vi "transform.vi"(9 "Demodulated signals":waveform(sgl)[][](array[waveform]), 11 "Configuration":T2) -> (0 "Sum amplitudes":sgl[][](array[numeric]), 1 "Match error":waveform(sgl)[](array[waveform]), 3 "XYZ out":T1(array[cluster]), 4 "Axis positions":sgl[][](array[numeric]))   [LabVIEW 2012]
uses:
  initialization/configuration.ctl
  initialization/asap_calibration.ctl
  <vilib>/Analysis/Matrix/Datatypes/RealMatrix.ctl
  <vilib>/Analysis/Matrix/NI_Matrix.lvlib
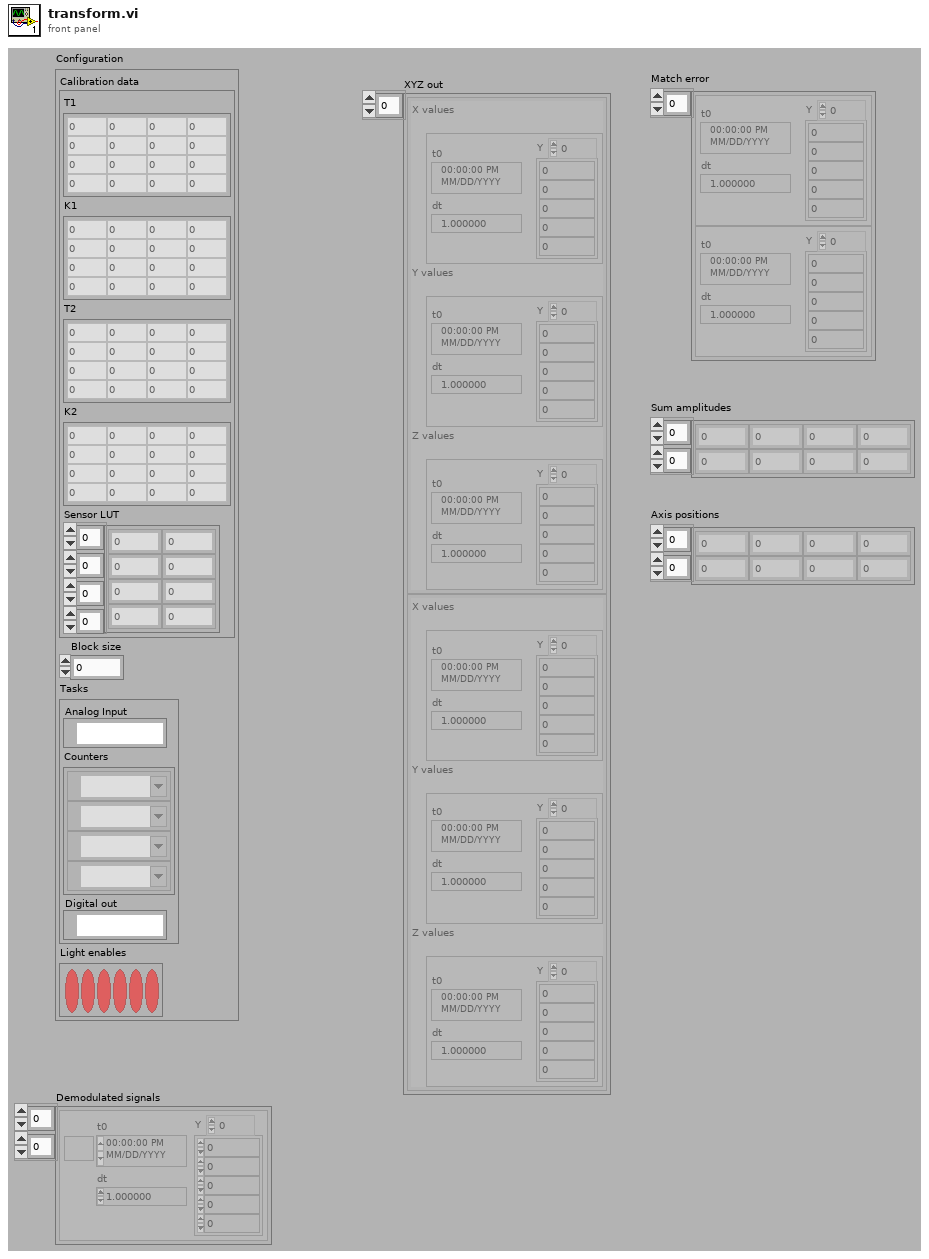
[diagram p1: front panel]
types:
  T1 = cluster{"X values":waveform(sgl), "Y values":waveform(sgl), "Z values":waveform(sgl)}[]
  T2 = typedef "configuration.ctl" = cluster{"Calibration data":T3, "Block size":i32, "Tasks":cluster{"Analog Input":refnum<k21>, "Counters":refnum<k21>[], "Digital out":refnum<k21>}, "Light enables":bool[]}
  T3 = typedef "asap_calibration.ctl" = cluster{"T1":T4, "K1":T4, "T2":T4, "K2":T4, "Sensor LUT":sgl[][][][]}
  T4 = typedef "NI_Matrix.lvlib/RealMatrix.ctl" = dbl[][]
  T5 = cluster{"X values":waveform(dbl), "Y values":waveform(dbl), "Z values":waveform(dbl)}
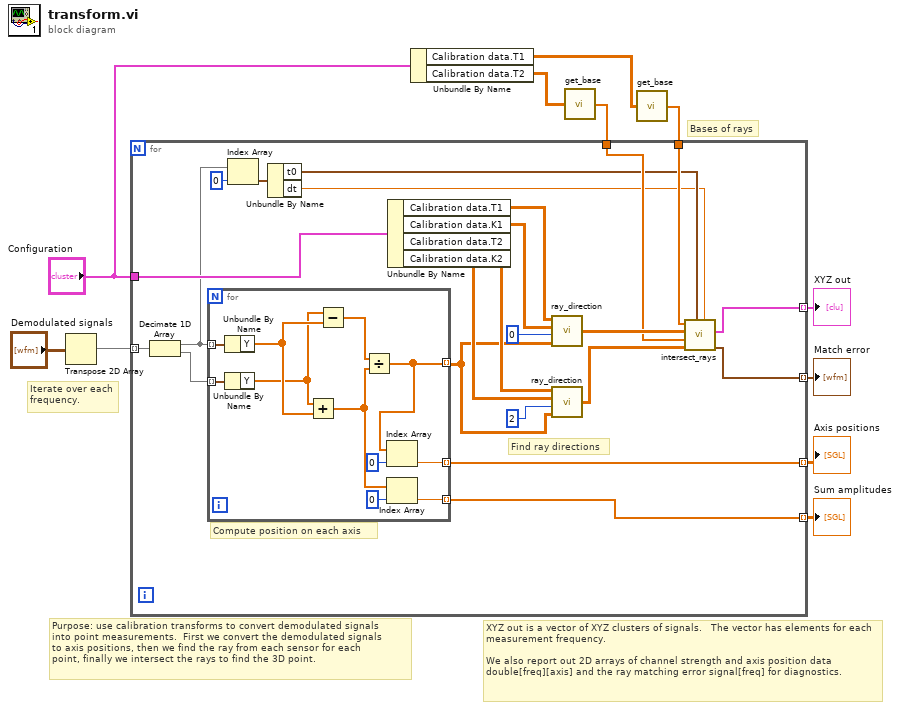
[diagram p0: block diagram]
diagram:
  # "Bases of rays"
  # "Purpose: use calibration transforms to convert demodulated signals\ninto point measurements.  First we convert the demodulated signals\nto axis positions, then we find the ray from each sensor for each\npoint, finally we intersect the rays to find the 3D point."
  # "XYZ out is a vector of XYZ clusters of signals.   The vector has elements for each\nmeasurement frequency. \n\nWe also report out 2D arrays of channel strength and axis position data double[freq][axis] and the ray matching error signal[freq] for diagnostics."
  # "Iterate over each\nfrequency."
  n1 = Transpose 2D Array(2D array="Demodulated signals") -> (transposed array=w10:waveform(sgl)[][])
  n2 = Unbundle By Name("Configuration") -> ("Calibration data.T1"=w5:T4, "Calibration data.T2"=w3:T4)
  n3 = call "get_base.vi"("T"=w3) -> ("Array"=w2:dbl[])
  n4 = call "get_base.vi"("T"=w5) -> ("Array"=w4:dbl[])
  n5 = for {
    tunnel: w10 -> [w34] mode=indexing
    tunnel: "Configuration" -> [w31]
    tunnel: [w32] -> w9 mode=indexing
    tunnel: w4 -> [w20]
    tunnel: w2 -> [w18]
    tunnel: [w14] -> w7 mode=indexing
    tunnel: [w13] -> w6 mode=indexing
    tunnel: [w12] -> w1 mode=indexing
    # "Find ray directions"
    # "Compute position on each axis"
    n6 = Decimate 1D Array(w34) -> (w30:waveform(sgl)[], w33:waveform(sgl)[])
    n7 = for {
      tunnel: [w36] -> w21 mode=indexing
      tunnel: w30 -> [w44] mode=indexing
      tunnel: w33 -> [w43] mode=indexing
      tunnel: [w40] -> w32 mode=indexing
      tunnel: [w35] -> w12 mode=indexing
      n8 = Unbundle By Name(w44) -> ("Y"=w39:sgl[])
      n9 = Unbundle By Name(w43) -> ("Y"=w38:sgl[])
      n10 = Add(x=w38, y=w39) -> (x+y=w42:sgl[])
      n11 = Subtract(x=w38, y=w39) -> (x-y=w45:sgl[])
      n12 = Divide(x=w45, y=w42) -> (x/y=w36:sgl[])
      n13 = Index Array(array=w36, index=0) -> (element=w35:sgl)
      n14 = Index Array(array=w42, index=0) -> (element=w40:sgl)
    }
    n15 = Index Array(array=w30, index=0) -> (element=w28:waveform(sgl))
    n16 = Unbundle By Name(w28) -> ("t0"=w16:timestamp, "dt"=w15:dbl)
    n17 = Unbundle By Name(w31) -> ("Calibration data.T1"=w27:T4, "Calibration data.K1"=w26:T4, "Calibration data.T2"=w23:T4, "Calibration data.K2"=w22:T4)
    n18 = call "ray_direction.vi"("Axis positions"=w21, "first axis"=0 ("index"), "K"=w26, "T"=w27) -> ("Ray directions"=w19:T4)  [unwired: 2 out]
    n19 = call "ray_direction.vi"("Axis positions"=w21, "first axis"=2 ("index"), "K"=w22, "T"=w23) -> ("Ray directions"=w17:T4)  [unwired: 2 out]
    n20 = call "intersect_rays.vi"("dt"=w15, "t0"=w16, "Sensor 2 directions"=w17, "Sensor 2 base"=w18, "Sensor 1 directions"=w19, "Sensor 1 base"=w20) -> ("Match error"=w13:waveform(dbl), "XYZ"=w14:T5)  [unwired: 4 out]
  }
  "XYZ out" <- w7
  "Sum amplitudes" <- w9
  "Match error" <- w6
  "Axis positions" <- w1
